vi "Wiimote LEDs Read.vi"(8 "error in (no error)":errorcluster, 9 "Wiimote Player #":i32=1, 11 "LV WiiMote Interface In":T2) -> (0 "error out":errorcluster, 2 "Wiimote LEDs out":T1, 3 "LV WiiMote Interface out":T2)   [LabVIEW 2012, in "LV Wiimote Interface.lvclass"]
uses:
  LV Wiimote Interface.lvclass
  Controls/LV Wiimote Interface.ctl
  Controls/Wiimote LEDs.ctl
  C:/Program Files/National Instruments/LabVIEW 2012/vi.lib/LabVIEW Hacker/WiiMote/Dependencies/WiimoteLib.dll
  Program Files/National Instruments/LabVIEW 2012/vi.lib/LabVIEW Hacker/WiiMote/Dependencies/WiimoteLib.dll
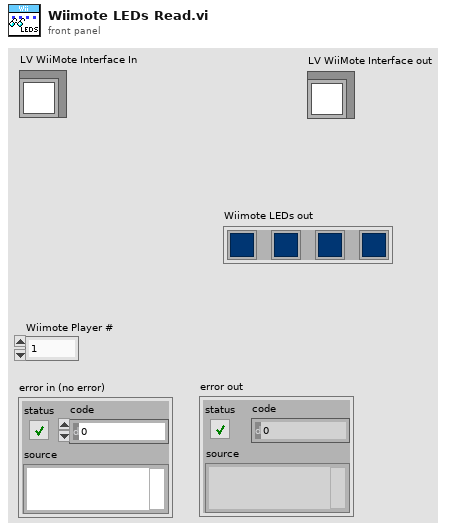
[diagram p1: front panel]
types:
  T1 = typedef "LV Wiimote Interface.lvclass/Wiimote LEDs.ctl" = cluster{"Wiimote LED":bool, "Wiimote LED 2":bool, "Wiimote LED 3":bool, "Wiimote LED 4":bool}
  T2 = typedef "LV Wiimote Interface.ctl" = refnum<class "LV Wiimote Interface.lvclass">
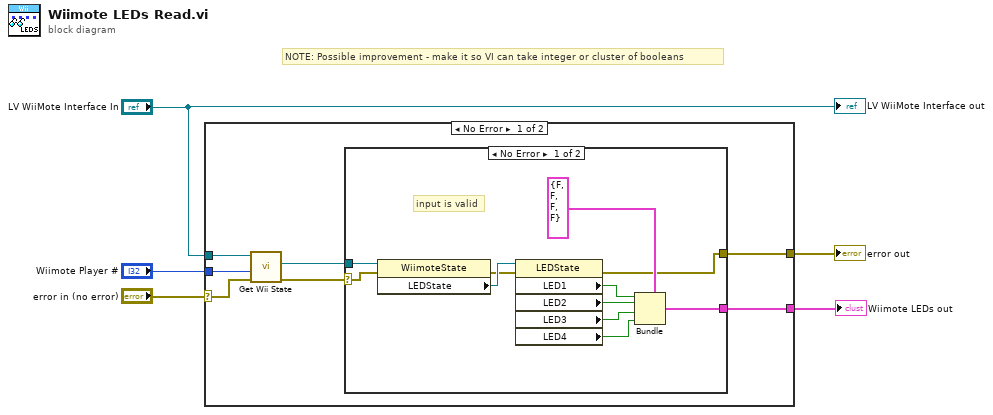
[diagram p0: block diagram]
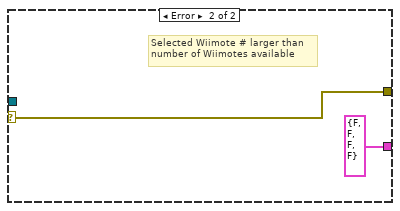
[diagram p2: hidden frame]
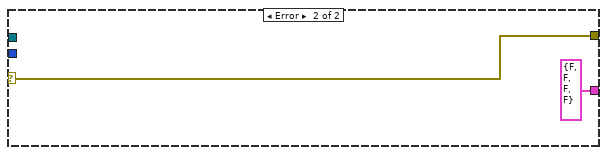
[diagram p3: hidden frame]
diagram:
  # "NOTE: Possible improvement - make it so VI can take integer or cluster of booleans"
  n1 = case shown="No Error" "error in (no error)" {
    selector: "error in (no error)" -> [w10 w27]
    tunnel: "LV WiiMote Interface In" -> [w12 _]
    tunnel: "Wiimote Player #" -> [w11 _]
    tunnel: [w7 w27] -> w3
    tunnel: [w6 T1 {"Wiimote LED"=FALSE, "Wiimote LED 2"=FALSE, "Wiimote LED 3"=FALSE, "Wiimote LED 4"=FALSE} ("Wiimote LEDs out")] -> w1
    frame No Error {
      n2 = call "Get Wii State.vi"("error in (no error)"=w10, "Wiimote Player #"=w11, "LV Wiimote Interface in"=w12) -> ("error out"=w9:errorcluster, "WiimoteState"=w8:refnum<k24>)  [unwired: 6 in, 1 out]
      n3 = case shown="No Error" w9 {
        selector: w9 -> [w22 w25]
        tunnel: [w13 w25] -> w7
        tunnel: w8 -> [w23 _]
        tunnel: [w14 T1 {"Wiimote LED"=FALSE, "Wiimote LED 2"=FALSE, "Wiimote LED 3"=FALSE, "Wiimote LED 4"=FALSE} ("Wiimote LEDs out")] -> w6
        frame No Error {
          # "input is valid"
          n4 = property class="WiimoteState"(reference=w23, error in=w22) -> (error out=w20:errorcluster, "LEDState"=w21:refnum<k24>)  [unwired: 1 out]
          n5 = property class="LEDState"(reference=w21, error in=w20) -> (error out=w13:errorcluster, "LED1"=w18:bool, "LED2"=w17:bool, "LED3"=w16:bool, "LED4"=w15:bool)  [unwired: 1 out]
          n6 = Bundle(cluster=T1 {"Wiimote LED"=FALSE, "Wiimote LED 2"=FALSE, "Wiimote LED 3"=FALSE, "Wiimote LED 4"=FALSE} ("Wiimote LEDs out"), "Wiimote LED"=w18, "Wiimote LED 2"=w17, "Wiimote LED 3"=w16, "Wiimote LED 4"=w15) -> (w14:T1)
        }
        frame Error {
          # "Selected Wiimote # larger than \nnumber of Wiimotes available"
        }
      }
    }
    frame Error {
    }
  }
  "error out" <- w3
  "Wiimote LEDs out" <- w1
  "LV WiiMote Interface out" <- "LV WiiMote Interface In"
